vi "3-lorentzian-heat-response -- analytic derivatives.vi"(0 "ζ":dbl(slide)=0.000285 min=0.0 max=0.3 step=1e-06 scale=0.01..10.0 scale format="%#_3p", 1 "T1":dbl(slide)=0.000285 min=0.0 max=0.3 step=1e-06 scale=0.01..10.0 scale format="%#_3p", 2 "τS":dbl(slide)=0.000285 min=0.0 max=0.3 step=1e-06 scale=0.01..10.0 scale format="%#_3p", 3 "τN":dbl(slide)=0.000285 min=0.0 max=0.3 step=1e-06 scale=0.01..10.0 scale format="%#_3p", 4 "τC":dbl(slide)=0.000285 min=0.0 max=0.3 step=1e-06 scale=0.01..10.0 scale format="%#_3p", 5 "κ0":dbl(slide)=0.000285 min=0.0 max=0.3 step=1e-06 scale=0.01..10.0 scale format="%#_3p", 7 "ω (rad/sec)":dbl=0.1 format="%#_10f", 8 "action":T1) -> (13 "R(ω)":cdb=0.1+0.0i format="%#_10f", 14 "d R(ω) / dζ":cdb=-1.0+0.0i, 15 "d R(ω) /  dT1":cdb=-1.0+0.0i, 16 "d R(ω) /  d τS":cdb=-1.0+0.0i, 17 "d R(ω) /  d τN":cdb=-1.0+0.0i, 18 "d R(ω) /  d τC":cdb=-1.0+0.0i, 19 "d R(ω) /  d κ0":cdb=-1.0+0.0i)   [LabVIEW 2020]
uses:
  3-lorentzian-heat-response action.ctl
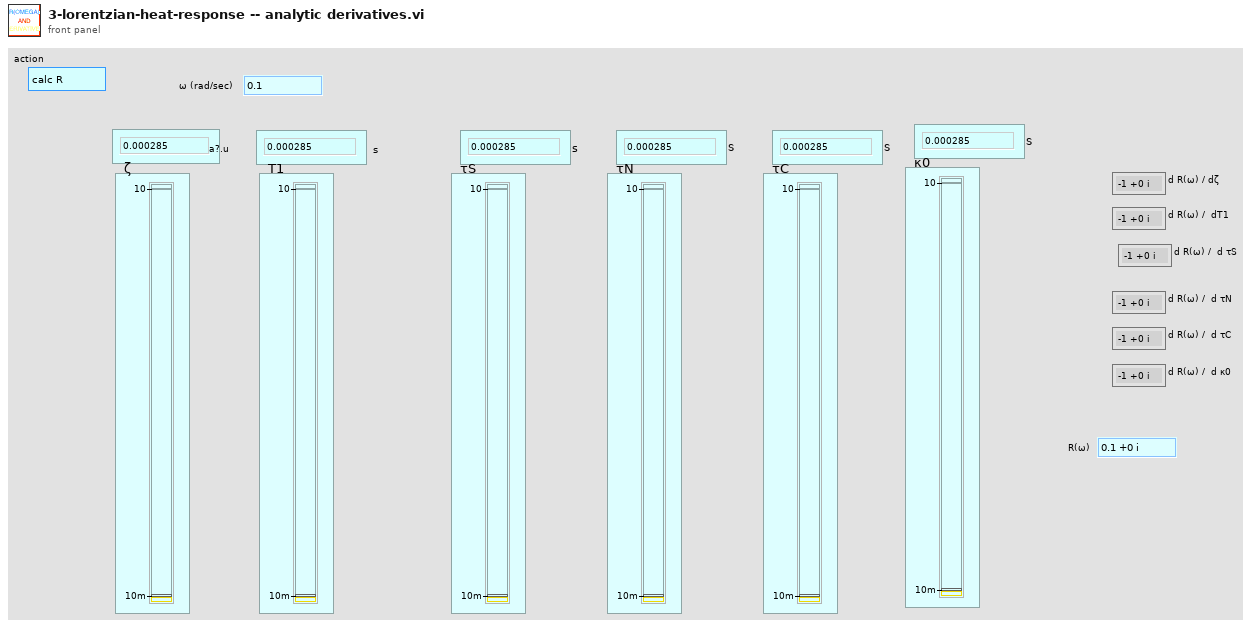
[diagram p1: front panel]
types:
  T1 = typedef "3-lorentzian-heat-response action.ctl" = enum16{"calc R", "create string", "calc m1m2m3", "dζ", "dT1", "dτS", "dτN", "dτC", "d-all", "dκ0"}
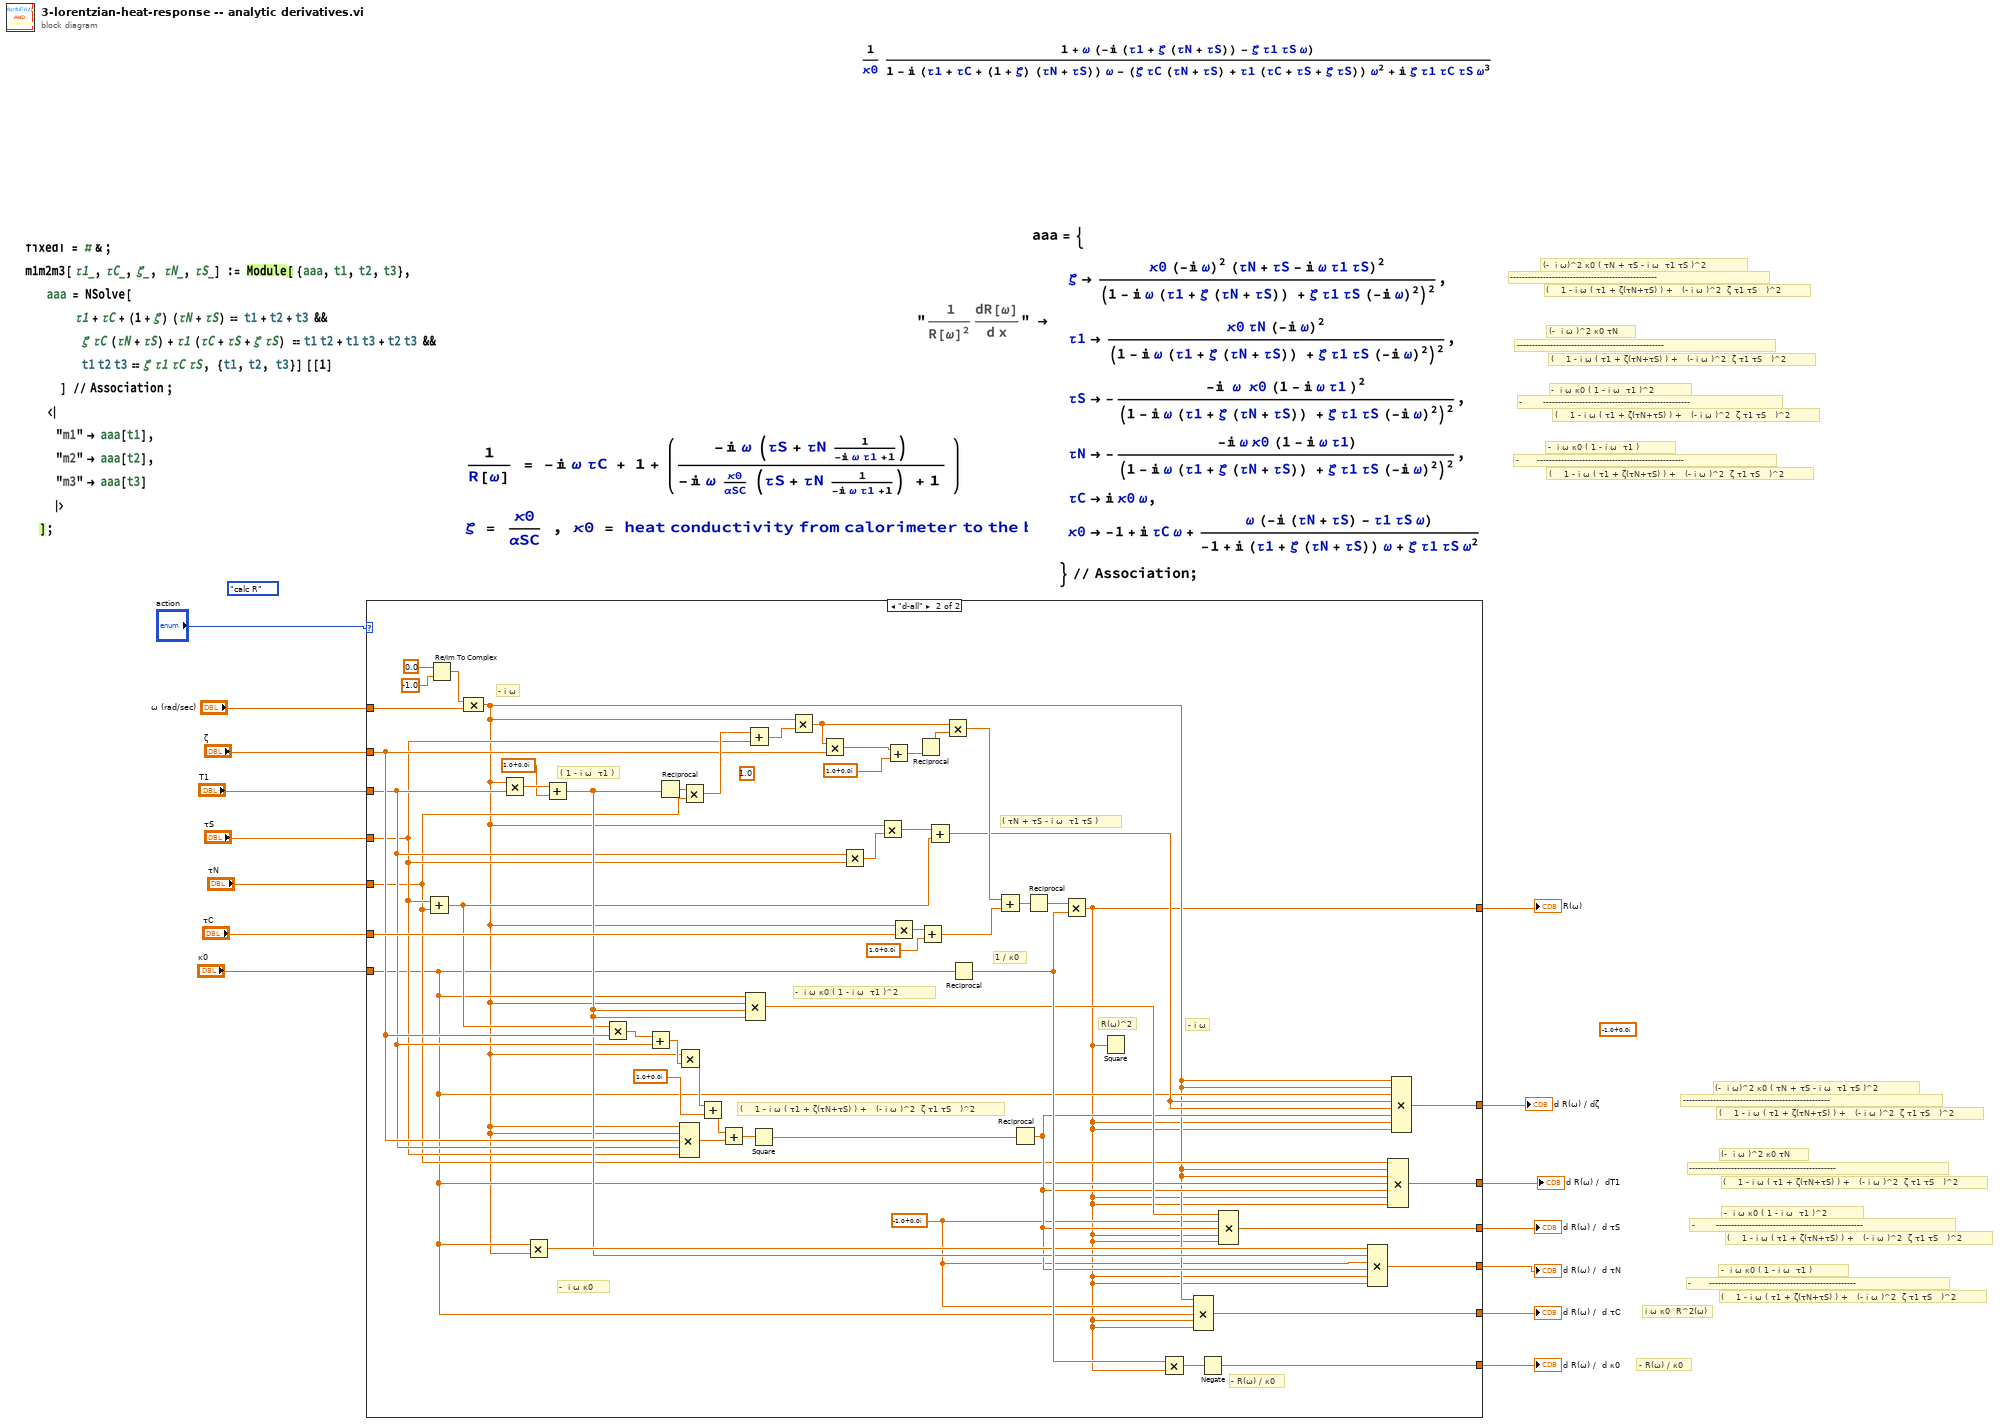
[diagram p0: block diagram]
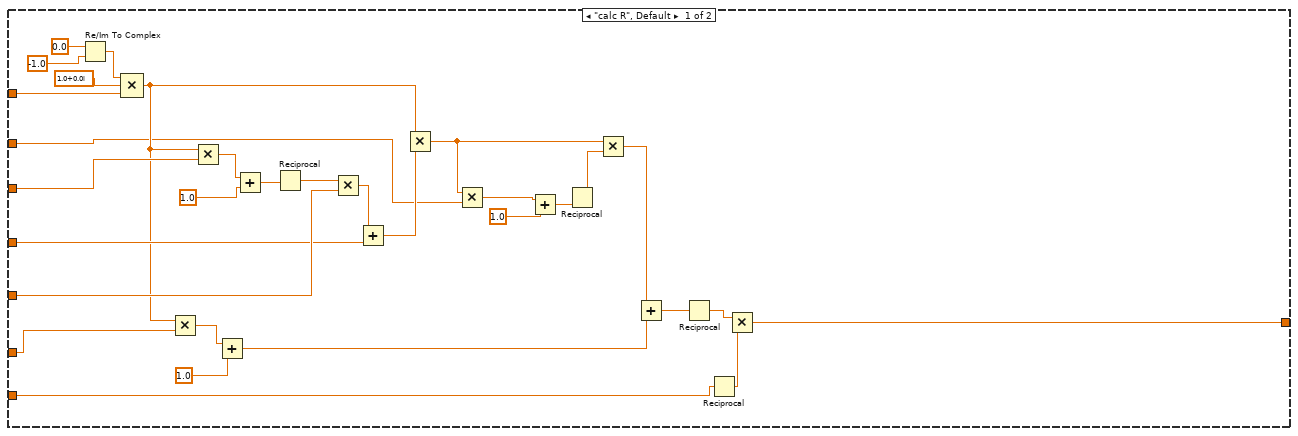
[diagram p2: hidden frame]
diagram:
  (unwired) cdb -1.0+0.0i ("value")
  (unwired) 3-lorentzian-heat-response_action."calc R" ("action")
  # "-------------------------------------------------"
  # "(-  i ω)^2 κ0 ( τN + τS - i ω  τ1 τS )^2"
  # "(    1 - i ω ( τ1 + ζ(τN+τS) ) +   (- i ω )^2  ζ τ1 τS   )^2"
  # "-------------------------------------------------"
  # "(-  i ω )^2 κ0 τN"
  # "(    1 - i ω ( τ1 + ζ(τN+τS) ) +   (- i ω )^2  ζ τ1 τS   )^2"
  # "-      -------------------------------------------------"
  # "-  i ω κ0 ( 1 - i ω  τ1 )"
  # "(    1 - i ω ( τ1 + ζ(τN+τS) ) +   (- i ω )^2  ζ τ1 τS   )^2"
  # "-       -------------------------------------------------"
  # "-  i ω κ0 ( 1 - i ω  τ1 )^2"
  # "(    1 - i ω ( τ1 + ζ(τN+τS) ) +   (- i ω )^2  ζ τ1 τS   )^2"
  # "-------------------------------------------------"
  # "(-  i ω)^2 κ0 ( τN + τS - i ω  τ1 τS )^2"
  # "(    1 - i ω ( τ1 + ζ(τN+τS) ) +   (- i ω )^2  ζ τ1 τS   )^2"
  # "-------------------------------------------------"
  # "(-  i ω )^2 κ0 τN"
  # "(    1 - i ω ( τ1 + ζ(τN+τS) ) +   (- i ω )^2  ζ τ1 τS   )^2"
  # "-      -------------------------------------------------"
  # "-  i ω κ0 ( 1 - i ω  τ1 )"
  # "(    1 - i ω ( τ1 + ζ(τN+τS) ) +   (- i ω )^2  ζ τ1 τS   )^2"
  # "-       -------------------------------------------------"
  # "-  i ω κ0 ( 1 - i ω  τ1 )^2"
  # "(    1 - i ω ( τ1 + ζ(τN+τS) ) +   (- i ω )^2  ζ τ1 τS   )^2"
  # "i ω κ0  R^2(ω)"
  # "- R(ω) / κ0"
  n1 = case shown="\"d-all\"" "action" {
    tunnel: "τC" -> [w32 w92]
    tunnel: "ω (rad/sec)" -> [w35 w94]
    tunnel: "T1" -> [w34 w59]
    tunnel: "τN" -> [w40 w51]
    tunnel: "τS" -> [w38 w58]
    tunnel: "ζ" -> [w28 w70]
    tunnel: [w16 w47] -> w7
    tunnel: "κ0" -> [w19 w50]
    tunnel: [_ w79] -> w6
    tunnel: [_ w78] -> w5
    tunnel: [_ w64] -> w4
    tunnel: [_ w61] -> w3
    tunnel: [_ w60] -> w2
    tunnel: [_ w52] -> w1
    frame "calc R", Default {
      n2 = Re/Im To Complex(1:-1.0 ("y"), 2:0.0 ("x")) -> (0:w36:cdb)
      n3 = Compound Arithmetic op=MULTIPLY(w36, cdb 1.0+0.0i ("value"), w35) -> (w30:cdb)
      n4 = Multiply(x=w30, y=w32) -> (x*y=w31:cdb)
      n5 = Multiply(x=w30, y=w34) -> (x*y=w33:cdb)
      n6 = Add(x=w31, y=1.0) -> (x+y=w22:cdb)
      n7 = Add(x=w33, y=1.0) -> (x+y=w42:cdb)
      n8 = Reciprocal(x=w42) -> (1/x=w41:cdb)
      n9 = Multiply(x=w41, y=w40) -> (x*y=w39:cdb)
      n10 = Add(x=w39, y=w38) -> (x+y=w29:cdb)
      n11 = Multiply(x=w30, y=w29) -> (x*y=w24:cdb)
      n12 = Multiply(x=w24, y=w28) -> (x*y=w26:cdb)
      n13 = Add(x=w26, y=1.0) -> (x+y=w25:cdb)
      n14 = Reciprocal(x=w25) -> (1/x=w23:cdb)
      n15 = Multiply(x=w24, y=w23) -> (x*y=w21:cdb)
      n16 = Add(x=w21, y=w22) -> (x+y=w20:cdb)
      n17 = Reciprocal(x=w20) -> (1/x=w18:cdb)
      n18 = Reciprocal(x=w19) -> (1/x=w17:dbl)
      n19 = Multiply(x=w18, y=w17) -> (x*y=w16:cdb)
    }
    frame "d-all" {
      w48 = cdb -1.0+0.0i ("value")
      (unwired) 1.0
      # "( τN + τS - i ω  τ1 τS )"
      # "-  i ω κ0"
      # "( 1 - i ω  τ1 )"
      # "(    1 - i ω ( τ1 + ζ(τN+τS) ) +   (- i ω )^2  ζ τ1 τS   )^2"
      # "-  i ω κ0 ( 1 - i ω  τ1 )^2"
      # "- i ω"
      # "1 / κ0"
      # "- R(ω) / κ0"
      # "- i ω"
      # "R(ω)^2"
      n20 = Add(x=w58, y=w51) -> (x+y=w55:dbl)
      n21 = Re/Im To Complex(1:-1.0 ("y"), 2:0.0 ("x")) -> (0:w95:cdb)
      n22 = Compound Arithmetic op=MULTIPLY(w95, w94) -> (w49:cdb)
      n23 = Multiply(x=w49, y=w59) -> (x*y=w93:cdb)
      n24 = Multiply(x=w50, y=w49) -> (x*y=w63:cdb)
      n25 = Add(x=w93, y=cdb 1.0+0.0i ("value")) -> (x+y=w62:cdb)
      n26 = Multiply(x=w55, y=w70) -> (x*y=w74:dbl)
      n27 = Add(x=w74, y=w59) -> (x+y=w73:dbl)
      n28 = Reciprocal(x=w62) -> (1/x=w97:cdb)
      n29 = Multiply(x=w49, y=w73) -> (x*y=w72:cdb)
      n30 = Compound Arithmetic op=MULTIPLY(w49, w49, w70, w59, w58) -> (w68:cdb)
      n31 = Multiply(x=w97, y=w51) -> (x*y=w96:cdb)
      n32 = Add(x=w72, y=cdb 1.0+0.0i ("value")) -> (x+y=w69:cdb)
      n33 = Add(x=w69, y=w68) -> (x+y=w67:cdb)
      n34 = Add(x=w96, y=w58) -> (x+y=w90:cdb)
      n35 = Compound Arithmetic op=MULTIPLY(w50, w49, w62, w62) -> (w66:cdb)
      n36 = Square(x=w67) -> (x^2=w65:cdb)
      n37 = Multiply(x=w49, y=w90) -> (x*y=w87:cdb)
      n38 = Multiply(x=w87, y=w70) -> (x*y=w89:cdb)
      n39 = Multiply(x=w59, y=w58) -> (x*y=w57:dbl)
      n40 = Multiply(x=w49, y=w57) -> (x*y=w56:cdb)
      n41 = Add(x=w89, y=cdb 1.0+0.0i ("value")) -> (x+y=w88:cdb)
      n42 = Multiply(x=w49, y=w92) -> (x*y=w91:cdb)
      n43 = Reciprocal(x=w88) -> (1/x=w86:cdb)
      n44 = Add(x=w91, y=cdb 1.0+0.0i ("value")) -> (x+y=w85:cdb)
      n45 = Add(x=w56, y=w55) -> (x+y=w54:cdb)
      n46 = Multiply(x=w87, y=w86) -> (x*y=w84:cdb)
      n47 = Reciprocal(x=w50) -> (1/x=w81:dbl)
      n48 = Add(x=w84, y=w85) -> (x+y=w83:cdb)
      n49 = Reciprocal(x=w65) -> (1/x=w53:cdb)
      n50 = Reciprocal(x=w83) -> (1/x=w82:cdb)
      n51 = Multiply(x=w82, y=w81) -> (x*y=w47:cdb)
      n52 = Square(x=w47) -> ()  [unwired: 1 out]
      n53 = Multiply(x=w81, y=w47) -> (x*y=w80:cdb)
      n54 = Compound Arithmetic op=MULTIPLY(w49, w48, w50, w47, w47) -> (w78:cdb)
      n55 = Negate(x=w80) -> (-x=w79:cdb)
      n56 = Compound Arithmetic op=MULTIPLY(w66, w48, w53, w47, w47) -> (w64:cdb)
      n57 = Compound Arithmetic op=MULTIPLY(w63, w62, w48, w53, w47, w47) -> (w61:cdb)
      n58 = Compound Arithmetic op=MULTIPLY(w51, w49, w49, w50, w53, w47, w47) -> (w60:cdb)
      n59 = Compound Arithmetic op=MULTIPLY(w49, w49, w50, w54, w54, w53, w47, w47) -> (w52:cdb)
    }
  }
  "R(ω)" <- w7
  "d R(ω) /  d κ0" <- w6
  "d R(ω) /  d τC" <- w5
  "d R(ω) /  d τS" <- w4
  "d R(ω) /  d τN" <- w3
  "d R(ω) /  dT1" <- w2
  "d R(ω) / dζ" <- w1
